vi "verif_time.vi"(8 "error in (no error)":errorcluster, 11 "State Machine in":refnum<class "State Machine.lvclass">) -> (0 "error out":errorcluster, 3 "State Machine out":refnum<class "State Machine.lvclass">)   [LabVIEW 2018, in "State Machine.lvclass"]
doc: "Este VI monitora se o tempo de uma dada ação foi excedido."
uses:
  State Machine.lvclass
  State Machine.lvclass/State Machine.ctl
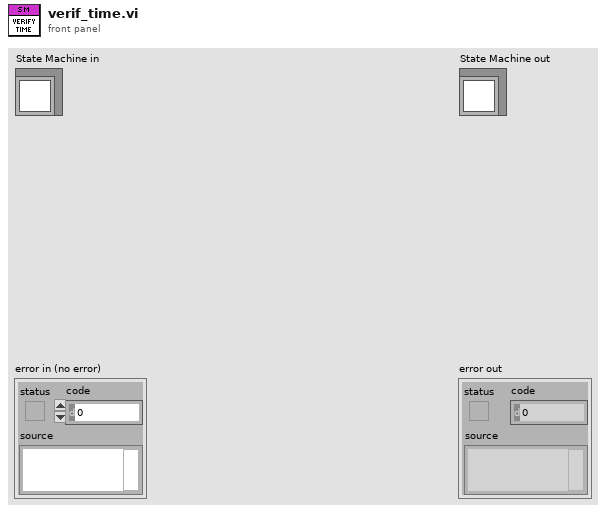
[diagram p1: front panel]
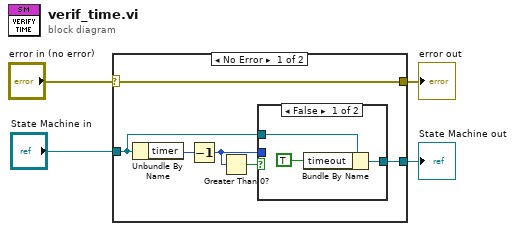
[diagram p0: block diagram]
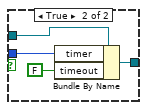
[diagram p2: hidden frame]
diagram:
  n1 = case shown="No Error" "error in (no error)" {
    selector: "error in (no error)" -> [w10 w19]
    tunnel: [w10 w19] -> w2
    tunnel: [w9 w18] -> w3
    tunnel: "State Machine in" -> [w8 w18]
    frame No Error {
      n2 = Unbundle By Name(w8) -> ("timer"=w6:u32)
      n3 = Decrement(x=w6) -> (x-1=w5:u32)
      n4 = Greater Than 0?(x=w5) -> (x > 0?=w7:bool)
      n5 = case shown="False" w7 {
        tunnel: [w11 w17] -> w9
        tunnel: w8 -> [w12 w16]
        tunnel: w5 -> [_ w14]
        frame False {
          n6 = Bundle By Name(cluster=w12, "timeout"=TRUE) -> (w11:refnum<class "State Machine.lvclass">)
        }
        frame True {
          n7 = Bundle By Name(cluster=w16, "timer"=w14, "timeout"=FALSE) -> (w17:refnum<class "State Machine.lvclass">)
        }
      }
    }
    frame Error {
    }
  }
  "error out" <- w2
  "State Machine out" <- w3
